vi "Waveform.vi"(0 "Top":i16, 1 "Left":i16, 2 "Time (ms)":u32=1000, 3 "error in":errorcluster) -> (10 "error out":errorcluster)   [LabVIEW 2012]
panel:
  out "Audio Signal":waveform(dbl)(graph)
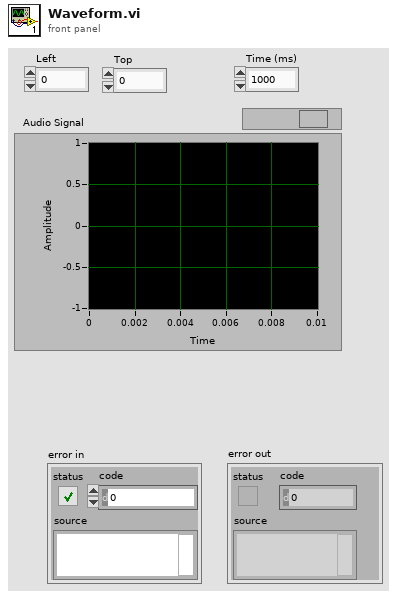
[diagram p1: front panel]
types:
  T1 = typedef "LVRectTypeDef.ctl" = cluster{"Left":i16, "Top":i16, "Right":i16, "Bottom":i16}
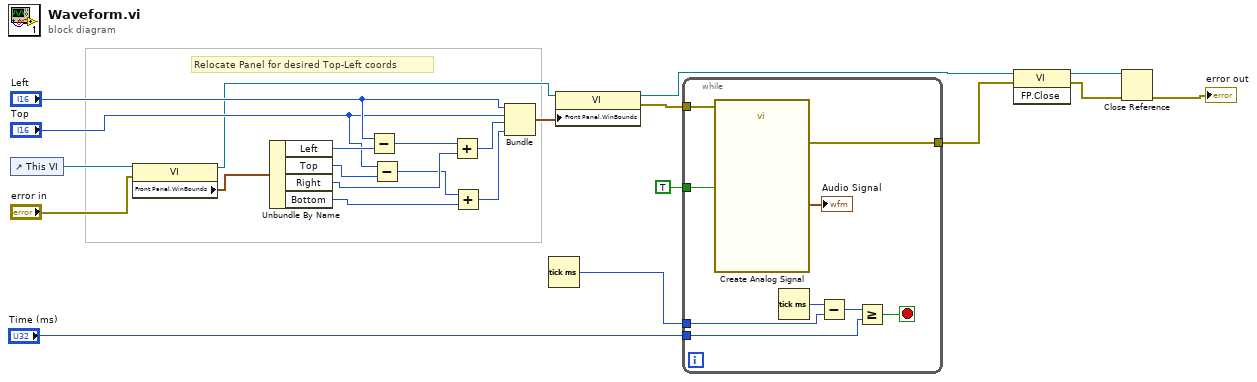
[diagram p0: block diagram]
diagram:
  # "Relocate Panel for desired Top-Left coords"
  n1 = control-ref of="This VI"() -> (w17:refnum<vi>)
  n2 = property class="VI"(reference=w17, error in="error in") -> (reference out=w2:refnum<vi>, "Front Panel.WinBounds"=w16:T1)  [unwired: 1 out]
  n3 = Unbundle By Name(w16) -> ("Left"=w14:i16, "Top"=w12:i16, "Right"=w10:i16, "Bottom"=w7:i16)
  n4 = Subtract(x="Left", y=w14) -> (x-y=w11:i16)
  n5 = Subtract(x="Top", y=w12) -> (x-y=w8:i16)
  n6 = Add(x=w11, y=w10) -> (x+y=w9:i16)
  n7 = Add(x=w8, y=w7) -> (x+y=w6:i16)
  n8 = Bundle("Left"="Left", "Top"="Top", w9, w6) -> (w5:cluster{"Left":i16, "Top":i16, i16, i16})  [unwired: 1 in]
  n9 = Tick Count (ms)() -> (millisecond timer value=w24:u32)
  n10 = property class="VI"(reference=w2, "Front Panel.WinBounds"=w5) -> (reference out=w1:refnum<vi>, error out=w3:errorcluster)  [unwired: 1 in]
  n11 = while {
    tunnel: [w33] -> w20
    tunnel: w24 -> [w31]
    tunnel: "Time (ms)" -> [w29]
    tunnel: TRUE -> [w27]
    tunnel: w3 -> [w25]
    stop <- w28 stop-if-true
    n12 = call "Create Analog Signal"("error in"=w25, "reset"=w27) -> ("multi-tone"=→"Audio Signal":waveform(dbl), "error out"=w33:errorcluster)  [unwired: 13 in, 3 out]
    n13 = Tick Count (ms)() -> (millisecond timer value=w32:u32)
    n14 = Subtract(x=w32, y=w31) -> (x-y=w30:u32)
    n15 = Greater Or Equal?(x=w30, y=w29) -> (x >= y?=w28:bool)
  }
  n16 = invoke class="VI" method="FP.Close"(reference=w1, error in=w20) -> (reference out=w18:refnum<vi>, error out=w19:errorcluster)  [unwired: 1 in, 1 out]
  n17 = Close Reference(reference=w18, error in (no error)=w19) -> (error out=→"error out":errorcluster)
